vi "Test_acceptCommand_wait.vi"(8 "error in (no error)":errorcluster, 11 "command_wait_Ctl":T1) -> (0 "error out":errorcluster, 2 "function return":i32, 3 "command_wait_Ctl out":T1)   [LabVIEW 2016, in "SALLV_Test.lvlib"]
doc: "int Test_shm_acceptCommand_waitLV(Test_command_waitLV *command_wait_Ctl );"
uses:
  SALLV_Test.lvlib
  DataTypes/command_wait.ctl
  SALLV_Test.so
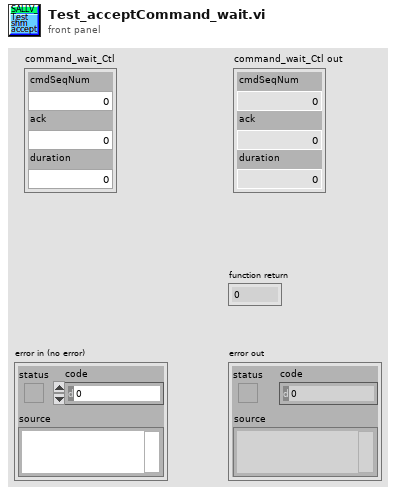
[diagram p1: front panel]
types:
  T1 = typedef "SALLV_Test.lvlib/command_wait.ctl" = cluster{"cmdSeqNum":i32, "ack":i32, "duration":dbl}
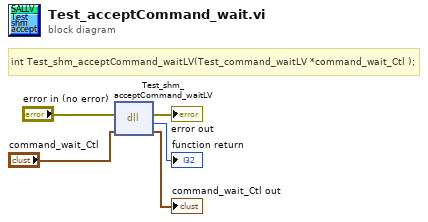
[diagram p0: block diagram]
diagram:
  # "int Test_shm_acceptCommand_waitLV(Test_command_waitLV *command_wait_Ctl );"
  n1 = dll-call lib="home/ccontaxis/Code/SALLV_Test/SALLV_Test.*" fn="Test_shm_acceptCommand_waitLV"(error in="error in (no error)", "command_wait_Ctl"="command_wait_Ctl") -> (error out=→"error out":errorcluster, →"function return":i32, "command_wait_Ctl"=→"command_wait_Ctl out":T1)  [unwired: 2 in, 1 out]
